vi "GetHelp.vi"(11 "SaveForPrevious in":refnum<class "SaveForPrevious.lvclass">) -> (2 "Help":string, 3 "SaveForPrevious out":refnum<class "SaveForPrevious.lvclass">)   [LabVIEW 2014, in "SaveForPrevious.lvclass"]
uses:
  SaveForPrevious.lvclass
panel:
  in  "HelpText":string="LabVIEWCLI -OperationName SaveForPrevious -SourceDirectory <path of directory to save>  -Version <version files should be saved in>  [-Overwrite <whether to overwrite the source files>]  [-OutputDirectory <path of newly saved files>]  [-Password <password for VIs>]\n\n -SourceDirectory : Specifies the full path to the location of the source to be saved for a previous version. This can be a directory or LLB.\n -Version : Specifies the previous LabVIEW version to save the files in. The oldest supported version is 8.0. An example would be 14.0 for LabVIEW 2014.\n -Overwrite : Specifies if the source files should be overwritten by the newly saved files. If false or not specified, output will be placed in -OutputDirectory or a new directory next to the -SourceDirectory.\n -OutputDirectory : Specifies the full path to the desired output location of the newly saved files. If -Overwrite is true, this parameter is ignored.\n -Password : Specifies a password to be used for opening the references to the VIs to be saved.\n"
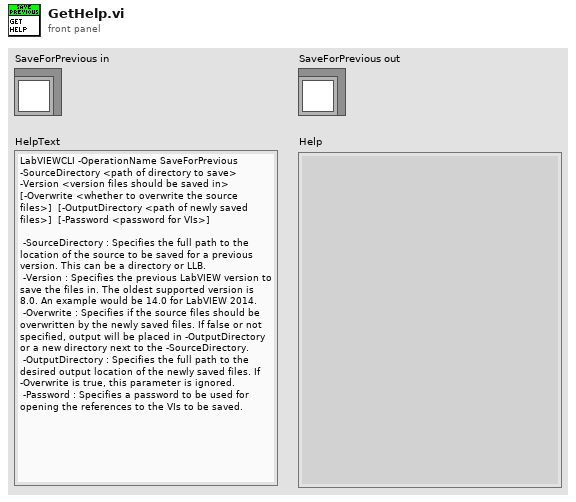
[diagram p1: front panel]
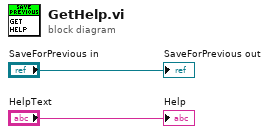
[diagram p0: block diagram]
diagram:
  "SaveForPrevious out" <- "SaveForPrevious in"
  "Help" <- "HelpText"
